vi "LWXPS_GetXVelParams.vi"(0 "XPS Reference IN":refnum<k24>, 11 "LabVIEW error IN":errorcluster) -> (4 "XPS Reference OUT":refnum<k24>, 6 "Returned error code":i32, 8 "Velocity X":dbl, 10 "XPS Error String":string, 15 "LabVIEW error OUT":errorcluster)   [LabVIEW 2014]
uses:
  D:/XPSQ8_LabView_Library/Development/Source/Dll/Newport.XPS.CommandInterface.dll
  Dll/Newport.XPS.CommandInterface.dll
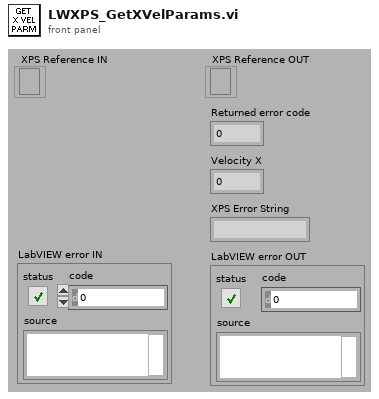
[diagram p1: front panel]
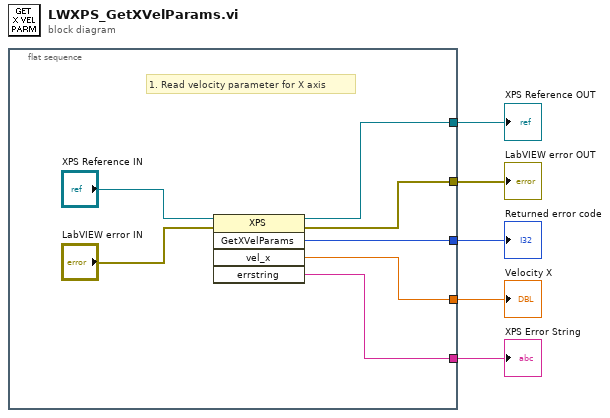
[diagram p0: block diagram]
diagram:
  n1 = flat-sequence {
    tunnel: [w7] -> w5
    tunnel: [w11] -> w4
    tunnel: [w9] -> w3
    tunnel: [w8] -> w2
    tunnel: [w6] -> w1
    frame #0 {
      # "1. Read velocity parameter for X axis"
      n2 = invoke class="XPS" method="GetXVelParams"(reference="XPS Reference IN", error in="LabVIEW error IN") -> (reference out=w7:refnum<k24>, error out=w11:errorcluster, "GetXVelParams"=w9:i32, "vel_x"=w6:dbl, "errstring"=w8:string)  [unwired: 3 in]
    }
  }
  "XPS Reference OUT" <- w5
  "LabVIEW error OUT" <- w4
  "Returned error code" <- w3
  "XPS Error String" <- w2
  "Velocity X" <- w1
